vi "Easy Data.vi"() -> ()   [LabVIEW 2012]
doc: "This revision adds the ability to acquire data from a local computer running Dataserver software. It is also possible to type in the address for a new Dataserver computer that is not listed on the ceeserver webpage."
uses:
  support/method.ctl
  DataServer/command cluster.ctl
  DataServer/command.ctl
  DAQ configuration/Sensor array.ctl
  DAQ configuration/channel identifier.ctl
  toolbar icons/data not logging.ctl
  toolbar icons/open configuration.ctl
  DAQ configuration/stream state.ctl
  TCP DAQ/Set.ctl
  TCP DAQ/clear offset.ctl
  TCP DAQ/graph channel info.ctl
  toolbar icons/calibrator.ctl
  toolbar icons/log data.ctl
  toolbar icons/graph type.ctl
  TCP DAQ/zero.ctl
  toolbar icons/Data Source.ctl
  toolbar icons/help.ctl
  Process Controller 3.0/read-write.ctl
  Process Controller 3.0/ini interface.ctl
  DataServer/Server Stats.vi
  calibration/global scale array.vi
  <vilib>/Analysis/1siggen.llb/Ramp Pattern by Samples.vi
  <vilib>/Analysis/NI_AALBase.lvlib
panel:
  in  "Help":T1
  in  "Data Source":T2 caption="OK Button"
  in  "File Comment":bool
  in  "Freeze":bool
  in  "Clear":T3
  in  "Zero":T4
  in  "power user":bool
  out "XY Graph":T5(graph)
  in  "graph type":T6
  in  "Enable Logging data":T7
  in  "Calibrator":T8 caption="OK Button"
  out "digital display":dbl[](array[numeric]) format="%.2p"
  out "channel info":T9[](array[typedef])
  in  "calibration":T11(array[cluster])=[{"Set"=FALSE, "target value"=0.0, "Clear"=FALSE}, {"Set"=FALSE, "target value"=0.0, "Clear"=FALSE}, {"Set"=FALSE, "target value"=0.0, "Clear"=FALSE}, {"Set"=FALSE, "target value"=0.0, "Clear"=FALSE}, {"Set"=FALSE, "target value"=0.0, "Clear"=FALSE}, {"Set"=FALSE, "target value"=0.0, "Clear"=FALSE}, {"Set"=FALSE, "target value"=0.0, "Clear"=FALSE}, {"Set"=FALSE, "target value"=0.0, "Clear"=FALSE}, {"Set"=FALSE, "target value"=0.0, "Clear"=FALSE}, {"Set"=FALSE, "target value"=0.0, "Clear"=FALSE}, {"Set"=FALSE, "target value"=0.0, "Clear"=FALSE}, {"Set"=FALSE, "target value"=0.0, "Clear"=FALSE}] {"target value" format="%.1p"}
  in  "reset interval":dbl=1.0 min=1.0 format="%.1f"
  out "New Stream state":T12
  out "Stream state":T12
  in  "Display update frequency":ext=1.0 format="%.4f"
  out "Sampling data frequency":dbl
  in  "Open Configuration":T13
  out "file warning":T14
  in  "Sensor Array":T15
  out "scans acquired":u32
  out "seconds":u32
  out "data server address":string="calcium"
  in  "method":T17={"sampling interval"=0.1, "samples to average"=1, "data interval"=0.0, "stream data"=FALSE, "file path"=refnum, "command"={"command"=enum."Idle", "start time (ms)"=0, "Channel Indices"=[], "Scans per Sample"=1}} {"command"."Scans per Sample" min=1; "data interval" format="%.2f"; "samples to average" min=1 step=1; "sampling interval" format="%.2f"}
  in  "Data log status":bool
  in  "colors":u32[](array[colorbox])=[16711680, 16770090, 6487897, 16777215, 16753241, 16738047, 52479, 2556143, 16711680, 16770090, 7470980, 16777215, 16753241, 16738047, 52479, 2556143]
  out "error":errorcluster={"status"=FALSE, "code"=56, "source"="TCP Read in \u0000TCP read variable.vi->read Volts data fast.vi->Signal Monitor"}
  out "chart":sgl[][](graph)
  out "connection ID":refnum<k5>
  out "stop":bool=TRUE
  out "logging data to file:":path=path "C:/WINNT/Profiles/mlws/Desktop/50Hzjunk"
  # "current \nvalue"
  # "plot\ncolor"
  # "name"
  # "units"
  # "F1 toggles power user features"
  # "s"
  # "s"
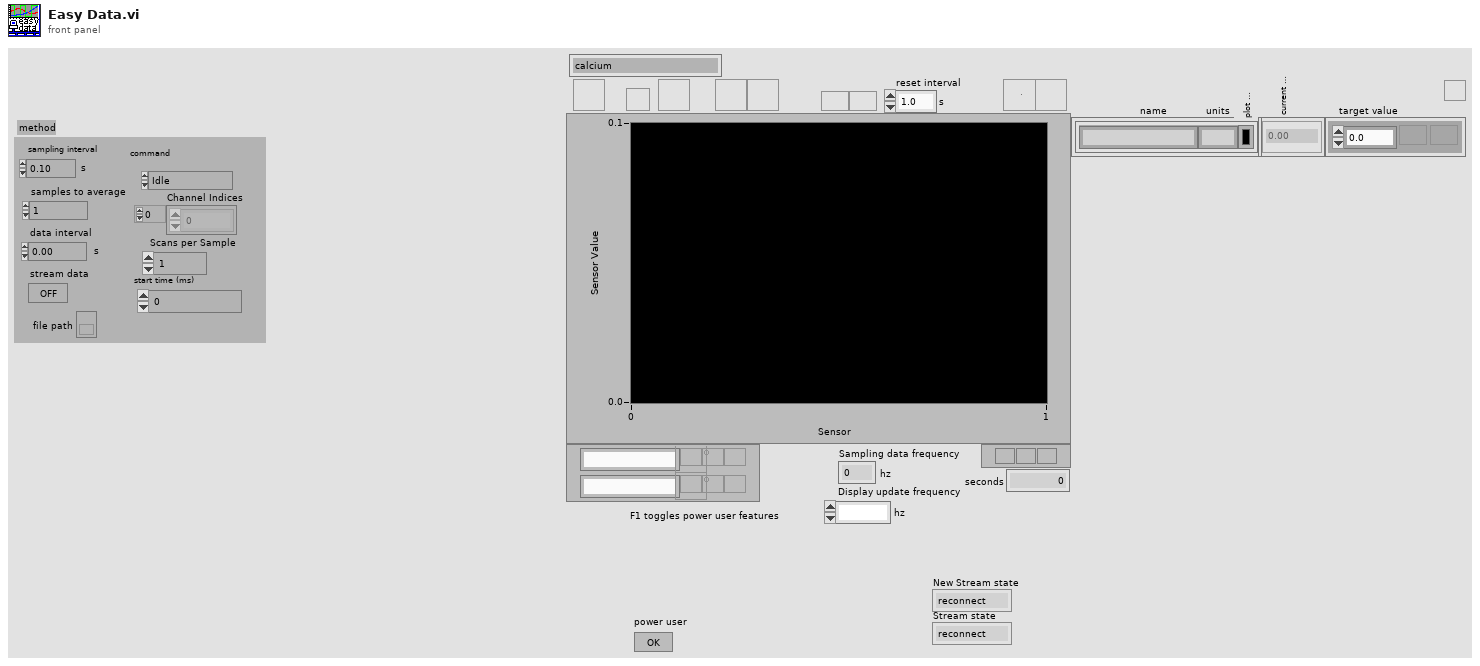
[diagram p1: front panel]
types:
  T1 = typedef "help.ctl" = bool
  T2 = typedef "Data Source.ctl" = bool
  T3 = typedef "clear offset.ctl" = bool
  T4 = typedef "zero.ctl" = bool
  T5 = cluster{"Ramp Pattern":dbl[], "last reading":sgl[]}
  T6 = typedef "graph type.ctl" = bool
  T7 = typedef "log data.ctl" = bool
  T8 = typedef "calibrator.ctl" = bool
  T9 = typedef "graph channel info.ctl" = cluster{"name":string, "units":string, "Color":u32}
  T10 = typedef "Set.ctl" = bool
  T11 = cluster{"Set":T10, "target value":dbl, "Clear":T3}[]
  T12 = typedef "stream state.ctl" = enum16{"reconnect", "Start", "Stream", "Clear", "Stop", "idle"}
  T13 = typedef "open configuration.ctl" = bool
  T14 = typedef "data not logging.ctl" = bool
  T15 = typedef "Sensor array.ctl" = T16[]
  T16 = typedef "channel identifier.ctl" = u16
  T17 = typedef "method.ctl" = cluster{"sampling interval":sgl, "samples to average":u32, "data interval":sgl, "stream data":bool, "file path":refnum<file>, "command":T18}
  T18 = typedef "command cluster.ctl" = cluster{"command":T19, "start time (ms)":u32, "Channel Indices":i32[], "Scans per Sample":i32}
  T19 = typedef "command.ctl" = enum16{"Idle", "Send Data", "Send 1 Scan", "Logoff"}
  T20 = typedef "ini interface.ctl" = enum16{"dataserver list", "dataserver", "com port", "stamp model", "Local Daq"}
  T21 = typedef "read-write.ctl" = enum16{"read", "write"}
  T22 = enum16{"Idle", "Send Data", "Send 1 Scan", "Logoff"}
  T23 = cluster{"Set":T10, "target value":dbl, "Clear":T3}
  T24 = typedef "Server stats.ctl" = cluster{"scan rate":dbl, "# connections":i32, "channel settings":cluster{"Name":string, "upper input limits":sgl, "lower input limits":sgl, "Location":string}[]}
  T25 = typedef "calib array.ctl" = T26[]
  T26 = typedef "conversion.ctl" = cluster{"conversion matrix":sgl[][], "units":string, "name":string, "scale type":T27, "offset (volts)":dbl, "second channel":i8, "correspondence table":T28, "offset (physical units)":dbl, "pH scale":T29, "D.O.":T30}
  T27 = typedef "scale type.ctl" = enum16{"Volts", "Polynomial", "Correspondence Table", "pH", "Dissolved Oxygen", "Quadratic"}
  T28 = typedef "correspondence table.ctl" = cluster{"physical units":dbl, "volts":dbl}[]
  T29 = typedef "pH scale.ctl" = cluster{"Buffers":cluster{"Buffer":dbl, "Calibrated":bool, "V/T":dbl}[], "Temperature":dbl}
  T30 = typedef "DO scale.ctl" = cluster{"Temperature":dbl, "K":dbl, "barometric pressure":dbl}
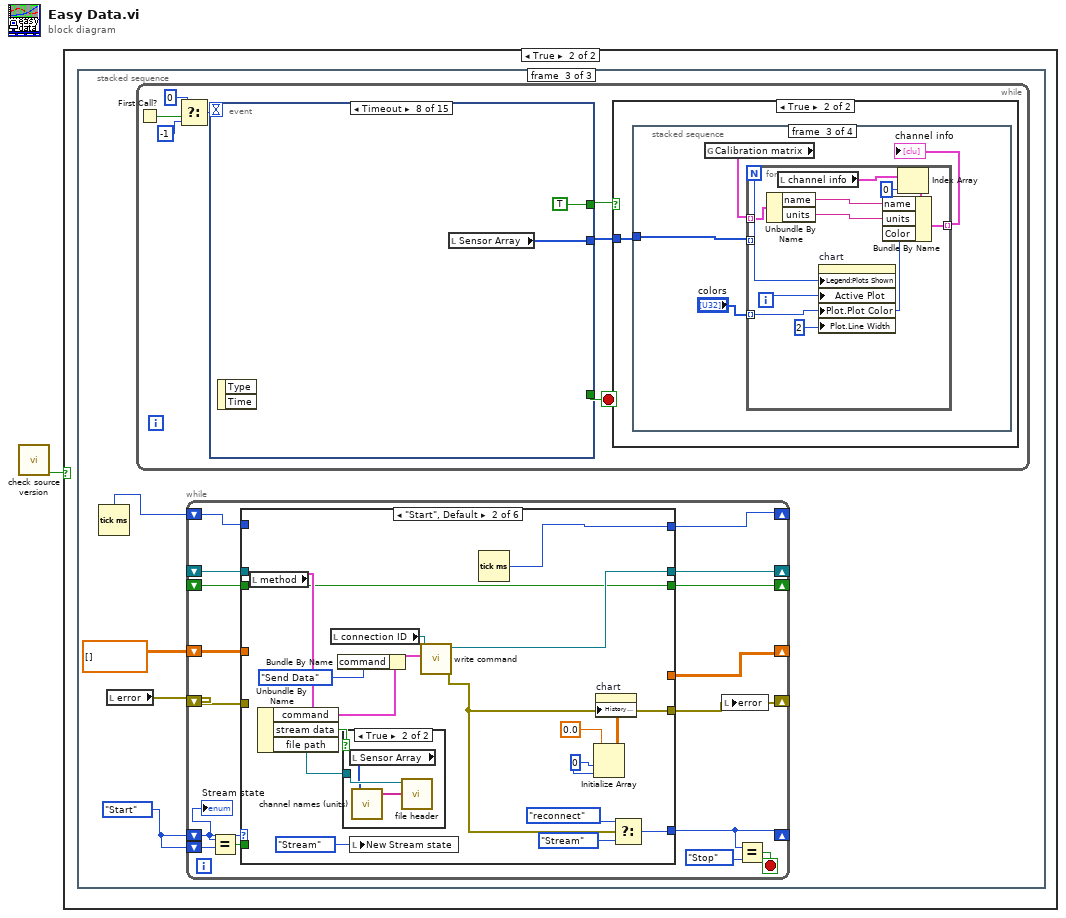
[diagram p0: block diagram]
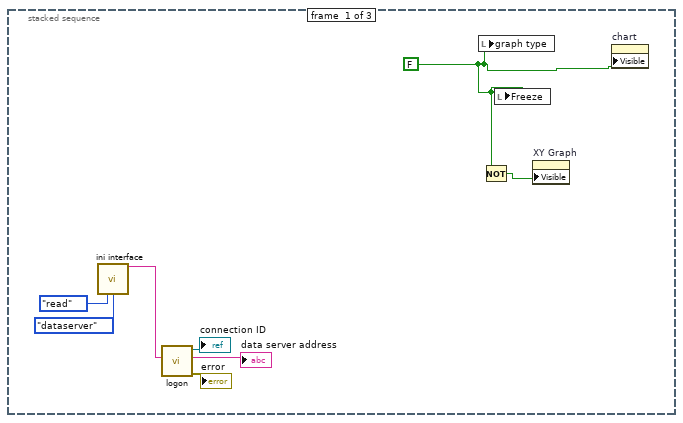
[diagram p3: hidden frame]
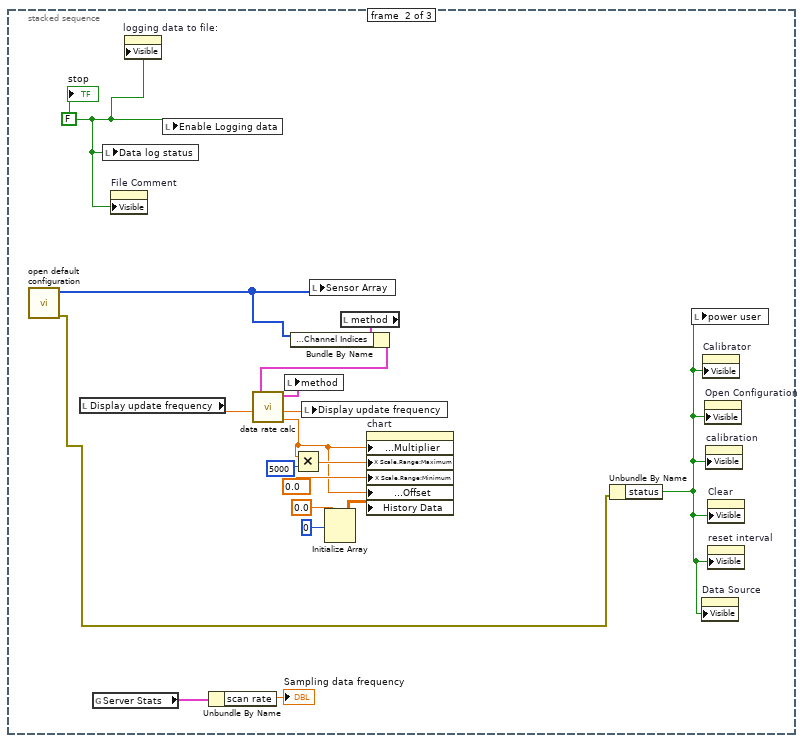
[diagram p4: hidden frame]
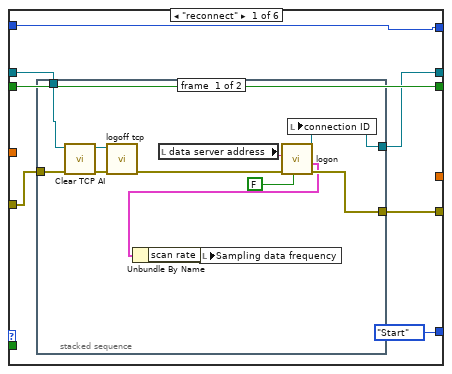
[diagram p5: hidden frame]
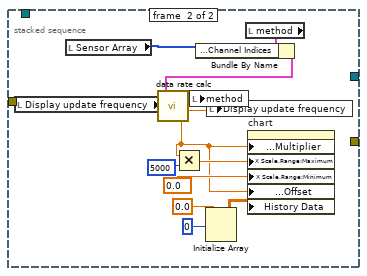
[diagram p6: hidden frame]
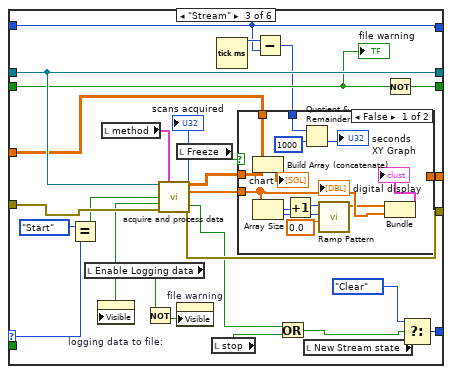
[diagram p8: hidden frame]
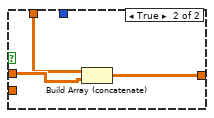
[diagram p9: hidden frame]
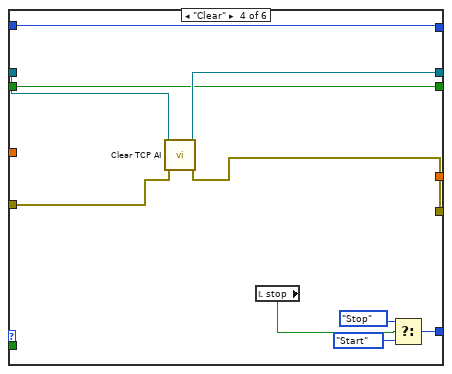
[diagram p10: hidden frame]
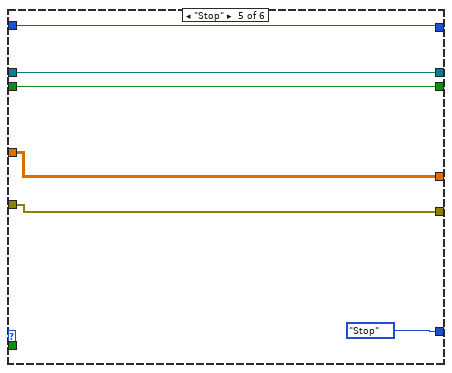
[diagram p11: hidden frame]
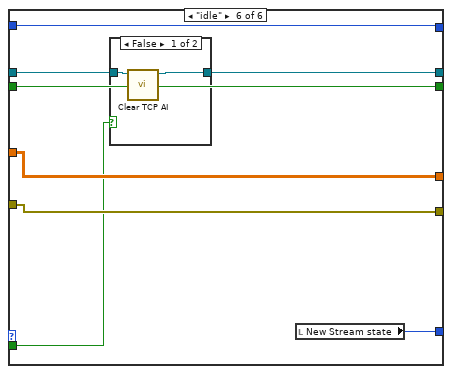
[diagram p12: hidden frame]
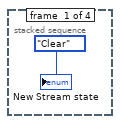
[diagram p15: hidden frame]
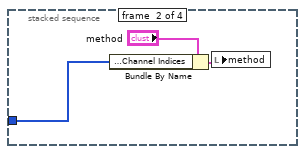
[diagram p16: hidden frame]
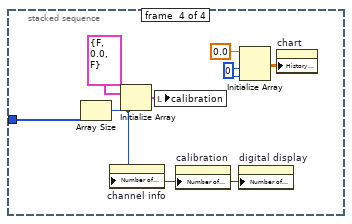
[diagram p17: hidden frame]
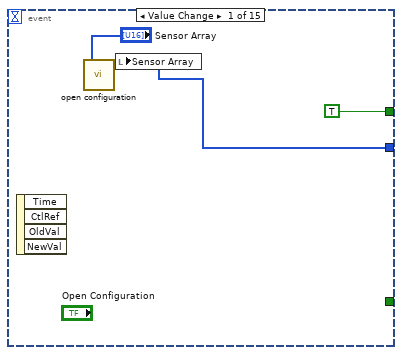
[diagram p18: hidden frame]
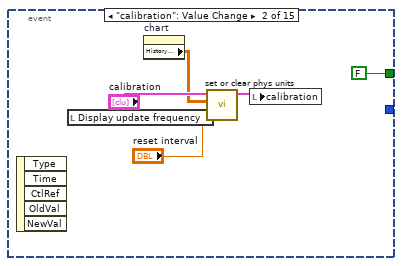
[diagram p19: hidden frame]
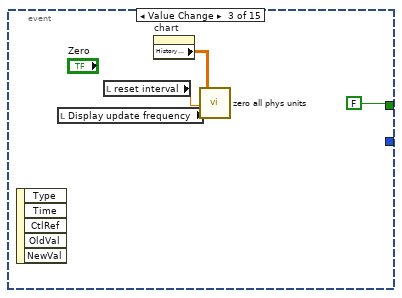
[diagram p20: hidden frame]
diagram:
  n1 = call "check source version.vi"() -> ("continue running?"=w1:bool)  [unwired: 2 in, 3 out]
  n2 = case shown="True" w1 {
    frame False {
    }
    frame True {
      n3 = stacked-sequence {
        frame #0 {
          w8 = T6 FALSE ("graph type")
          n4 = call "ini interface.vi"("direction"=read-write."read", "ini interface"=ini_interface."dataserver") -> ("dataserver out"=w2:string)  [unwired: 9 in, 4 out]
          n5 = call "logon.vi"("data server address in"=w2) -> ("error out"=→"error":errorcluster, "data server address"=→"data server address":string, "connection ID"=→"connection ID":refnum<k5>)  [unwired: 7 in, 1 out]
          n6 = local write "graph type"(w8) -> ()
          n7 = Not(x=w8) -> (.not. x?=w9:T6)
          n8 = local write "Freeze"(w8) -> ()
          n9 = property on="XY Graph" class="XYGraph (strict)"("Visible"=w9) -> ()  [unwired: 2 in, 2 out]
          n10 = property on="chart" class="WFChart (strict)"("Visible"=w8) -> ()  [unwired: 2 in, 2 out]
        }
        frame #1 {
          w23 = 0
          w25 = FALSE
          n11 = call "open default configuration.vi"() -> ("error out"=w12:errorcluster, "Sensor Array out"=w10:T15)  [unwired: 6 in]
          n12 = local read "Display update frequency"() -> (w14:ext)
          n13 = global read "Server Stats.vi" "Server Stats"() -> (w27:T24)
          n14 = local write "Data log status"(w25) -> ()
          n15 = property on="File Comment" class="Bool"("Visible"=w25) -> ()  [unwired: 2 in, 2 out]
          n16 = property on="logging data to file:" class="Path"("Visible"=w25) -> ()  [unwired: 2 in, 2 out]
          n17 = local write "Enable Logging data"(w25) -> ()
          n18 = Unbundle By Name(w27) -> ("scan rate"=→"Sampling data frequency":dbl)
          n19 = local write "Sensor Array"(w10) -> ()
          n20 = Initialize Array(sgl 0.0, w23, w23) -> (w17:sgl[][])
          n21 = local read "method"() -> (w16:T17)
          n22 = Bundle By Name(cluster=w16, "command.Channel Indices"=w10) -> (w15:T17)
          n23 = call "data rate calc.vi"("Data frequency"=w14, "method in"=w15) -> ("new data interval"=w18:sgl, "new data frequency"=w13:ext, "method out"=w19:T17)  [unwired: 2 in, 1 out]
          n24 = local write "method"(w19) -> ()
          n25 = Multiply(x=w18, y=5000) -> (x*y=w21:sgl)
          n26 = local write "Display update frequency"(w13) -> ()
          n27 = property on="chart" class="WFChart (strict)"("X Scale.Offset and Multiplier:Multiplier"=w18, "X Scale.Range:Maximum"=w21, "X Scale.Range:Minimum"=0.0, "X Scale.Offset and Multiplier:Offset"=w18, "History Data"=w17) -> ()  [unwired: 2 in, 2 out]
          n28 = Unbundle By Name(w12) -> ("status"=w11:bool)
          n29 = local write "power user"(w11) -> ()
          n30 = property on="Data Source" class="Bool"("Visible"=w11) -> ()  [unwired: 2 in, 2 out]
          n31 = property on="Calibrator" class="Bool"("Visible"=w11) -> ()  [unwired: 2 in, 2 out]
          n32 = property on="Open Configuration" class="Bool"("Visible"=w11) -> ()  [unwired: 2 in, 2 out]
          n33 = property on="calibration" class="Arr"("Visible"=w11) -> ()  [unwired: 2 in, 2 out]
          n34 = property on="Clear" class="Bool"("Visible"=w11) -> ()  [unwired: 2 in, 2 out]
          n35 = property on="reset interval" class="DigNum (strict)"("Visible"=w11) -> ()  [unwired: 2 in, 2 out]
          "stop" <- w25
        }
        frame #2 {
          w28 = stream_state."Start" ("Stream state")
          n36 = Tick Count (ms)() -> (millisecond timer value=w29:u32)
          n37 = local read "error"() -> (w31:errorcluster)
          n38 = while {
            stop <- w174 stop-if-true
            n39 = First Call?() -> (First Call?: T/F=w169:bool)
            n40 = Select(t=0, s=w169, f=-1) -> (s? t:f=w168:i32)
            n41 = event shown="[7] Timeout" {
              selector: _ -> [_ _ _ _ _ _ _ _ _ _ _ _ _ _ _]
              dyn-events: _ -> [_ _ _ _ _ _ _ _ _ _ _ _ _ _ _]
              timeout: w168 -> [_ _ _ _ _ _ _ _ _ _ _ _ _ _ _]
              tunnel: [_ _ _ _ _ _ w224 _ _ _ _ _ _ _ w293] -> w174
              tunnel: [w203 _ _ _ w218 _ _ w229 w231 _ _ _ _ _ _] -> w173
              tunnel: [TRUE FALSE FALSE _ TRUE _ w224 TRUE TRUE FALSE FALSE FALSE _ _ FALSE] -> w172
              event Value Change {
                n42 = event-data() -> ()  [unwired: 1 in, 4 out]
                n43 = call "open configuration.vi"("Sensor Array"="Sensor Array") -> ("Sensor Array out"=w203:T15)  [unwired: 5 in, 1 out]
                n44 = local write "Sensor Array"(w203) -> ()
              }
              event "calibration": Value Change {
                n45 = event-data() -> ()  [unwired: 1 in, 5 out]
                n46 = local read "Display update frequency"() -> (w208:ext)
                n47 = property on="chart" class="WFChart (strict)"() -> ("History Data"=w205:sgl[][])  [unwired: 2 in, 2 out]
                n48 = call "set or clear phys units.vi"("zero interval (s)"="reset interval", "Data frequency"=w208, "History Data"=w205, "calibration"="calibration") -> ("calibration out"=w207:T11)  [unwired: 3 in]
                n49 = local write "calibration"(w207) -> ()
              }
              event Value Change {
                n50 = event-data() -> ()  [unwired: 1 in, 5 out]
                n51 = local read "Display update frequency"() -> (w213:ext)
                n52 = local read "reset interval"() -> (w212:dbl)
                n53 = property on="chart" class="WFChart (strict)"() -> ("History Data"=w211:sgl[][])  [unwired: 2 in, 2 out]
                n54 = call "zero all phys units.vi"("zero interval (s)"=w213, "Data frequency"=w212, "History Data"=w211) -> ()  [unwired: 5 in]
              }
              event Value Change {
                n55 = event-data() -> ()  [unwired: 1 in, 5 out]
                n56 = local read "Sensor Array"() -> (w215:T15)
                n57 = for {
                  tunnel: w215 -> [_] mode=indexing
                  i -> [w216]
                  n58 = call "clear channel physical units.vi"("Index"=w216) -> ()  [unwired: 7 in]
                }
              }
              event Value Change {
                n59 = event-data() -> ()  [unwired: 1 in, 5 out]
                n60 = stacked-sequence {
                  tunnel: [_ w221] -> w218
                  frame #0 {
                    n61 = local write "New Stream state"(stream_state."idle" ("New Stream state")) -> ()
                  }
                  frame #1 {
                    n62 = local read "Sensor Array"() -> (w222:T15)
                    n63 = local read "data server address"() -> (w220:string)
                    n64 = call "Calibrator.vi"("data server address"=w220, "Channels"=w222) -> ("Ports out"=w221:T15)  [unwired: 6 in, 2 out]
                    n65 = local write "Sensor Array"(w221) -> ()
                  }
                }
              }
              event Value Change {
                n66 = event-data() -> ()  [unwired: 1 in, 6 out]
                n67 = call "Web Browser.vi"("URL"="http://ceeserver.cee.cornell.edu/mw24/Software/Easy Data.htm") -> ()  [unwired: 1 in]
              }
              event Value Change {
                w224 = FALSE
                n68 = event-data() -> ()  [unwired: 1 in, 6 out]
                n69 = stacked-sequence {
                  frame #0 {
                    n70 = call "Select server.vi"() -> ("DataSource"=w225:string)  [unwired: 5 in]
                    n71 = local write "data server address"(w225) -> ()
                    n72 = call "ini interface.vi"("dataserver"=w225, "direction"=read-write."write", "ini interface"=ini_interface."dataserver") -> ()  [unwired: 8 in, 5 out]
                  }
                  frame #1 {
                    n73 = local write "New Stream state"(stream_state."reconnect" ("New Stream state")) -> ()
                  }
                }
              }
              event Timeout {
                n74 = event-data() -> ()  [unwired: 1 in, 2 out]
                n75 = local read "Sensor Array"() -> (w229:T15)
              }
              event "Display update frequency": Value Change {
                w241 = 0
                n76 = event-data() -> ()  [unwired: 1 in, 5 out]
                n77 = local read "Sampling data frequency"() -> (w237:dbl)
                n78 = local read "method"() -> (w242:T17)
                n79 = In Range and Coerce(upper limit=w237, x="Display update frequency", lower limit=ext 0.01) -> (coerced(x)=w234:ext)  [unwired: 1 out]
                n80 = call "data rate calc.vi"("Data frequency"=w234, "method in"=w242) -> ("new data interval"=w233:sgl, "new data frequency"=w232:ext, "method out"=w243:T17)  [unwired: 2 in, 1 out]
                n81 = Initialize Array(w241, w241, w241) -> (w238:i32[][])
                n82 = local write "Display update frequency"(w232) -> ()
                n83 = Multiply(x=w233, y=5000) -> (x*y=w240:sgl)
                n84 = property on="chart" class="WFChart (strict)"("X Scale.Offset and Multiplier:Multiplier"=w233, "X Scale.Range:Maximum"=w240, "X Scale.Range:Minimum"=w241, "X Scale.Offset and Multiplier:Offset"=w233, "History Data"=w238) -> ()  [unwired: 2 in, 2 out]
                n85 = local write "method"(w243) -> ()
                n86 = local read "Sensor Array"() -> (w231:T15)
              }
              event Value Change {
                n87 = event-data() -> ()  [unwired: 1 in, 5 out]
                n88 = local read "Sensor Array"() -> (w245:T15)
                n89 = property on="file warning" class="Bool"("Visible"=FALSE) -> ()  [unwired: 2 in, 2 out]
                n90 = Not Equal?(x="Data log status", y="Enable Logging data") -> (x != y?=w250:T7)
                n91 = case shown="True" w250 {
                  tunnel: "Enable Logging data" -> [_ w252]
                  tunnel: w245 -> [_ w251]
                  frame False {
                  }
                  frame True {
                    n92 = case shown="True" w252 {
                      selector: w252 -> [w253 _]
                      tunnel: w251 -> [_ w258]
                      frame False {
                        n93 = local read "method"() -> (w255:T17)
                        n94 = local write "Data log status"(w253) -> ()
                        n95 = property on="logging data to file:" class="Path"("Visible"=w253) -> ()  [unwired: 2 in, 2 out]
                        n96 = Unbundle By Name(w255) -> ("file path"=w254:refnum<file>)
                        n97 = Bundle By Name(cluster=w255, "stream data"=w253, "file path"=refnum<k0> refnum) -> (w257:T17)
                        n98 = local write "method"(w257) -> ()
                        n99 = Close File(refnum=w254) -> ()  [unwired: 1 in, 2 out]
                        n100 = property on="File Comment" class="Bool"("Visible"=w253) -> ()  [unwired: 2 in, 2 out]
                      }
                      frame True {
                        n101 = call "Create xls File.vi"() -> ("error out"=w260:errorcluster, "path"=w259:path, "refnum"=w261:refnum<file>)  [unwired: 4 in, 1 out]
                        n102 = case shown="No Error" w260 {
                          tunnel: w261 -> [w264 _]
                          tunnel: w259 -> [w266 _]
                          tunnel: w258 -> [w262 _]
                          frame No Error {
                            n103 = Not A Number/Path/Refnum?(number/path/refnum=w264) -> (NaN/Path/Refnum?=w267:bool)
                            n104 = local read "method"() -> (w268:T17)
                            n105 = call "channel names (units).vi"("Sensor Array"=w262) -> ("channel strings"=w265:string[])  [unwired: 4 in]
                            n106 = Bundle By Name(cluster=w268, "stream data"=TRUE, "file path"=w264) -> (w269:T17)
                            n107 = Not(x=w267) -> (.not. x?=w263:bool)
                            n108 = local write "Enable Logging data"(w263) -> ()
                            n109 = local write "Data log status"(w263) -> ()
                            n110 = call "file header.vi"("channel strings"=w265, "refnum"=w264) -> ()  [unwired: 9 in, 1 out]
                            n111 = property on="logging data to file:" class="Path"("Visible"=w263) -> ()  [unwired: 2 in, 2 out]
                            n112 = local write "method"(w269) -> ()
                            n113 = property on="File Comment" class="Bool"("Visible"=w263) -> ()  [unwired: 2 in, 2 out]
                            "logging data to file:" <- w266
                          }
                          frame Error {
                            w271 = FALSE
                            n114 = local write "Enable Logging data"(w271) -> ()
                            n115 = local write "Data log status"(w271) -> ()
                            n116 = property on="logging data to file:" class="Path"("Visible"=w271) -> ()  [unwired: 2 in, 2 out]
                            n117 = property on="File Comment" class="Bool"("Visible"=w271) -> ()  [unwired: 2 in, 2 out]
                          }
                        }
                      }
                    }
                  }
                }
              }
              event Value Change {
                n118 = event-data() -> ()  [unwired: 1 in, 5 out]
                n119 = Not(x="graph type") -> (.not. x?=w272:T6)
                n120 = Not(x=w272) -> (.not. x?=w275:T6)
                n121 = property on="XY Graph" class="XYGraph (strict)"("Visible"=w272) -> ()  [unwired: 2 in, 2 out]
                n122 = property on="chart" class="WFChart (strict)"("Visible"=w275) -> ()  [unwired: 2 in, 2 out]
              }
              event "power user": Value Change {
                n123 = event-data() -> ()  [unwired: 1 in, 5 out]
                n124 = property on="calibration" class="Arr"("Visible"="power user") -> ()  [unwired: 2 in, 2 out]
                n125 = property on="Calibrator" class="Bool"("Visible"="power user") -> ()  [unwired: 2 in, 2 out]
                n126 = property on="Open Configuration" class="Bool"("Visible"="power user") -> ()  [unwired: 2 in, 2 out]
                n127 = property on="Clear" class="Bool"("Visible"="power user") -> ()  [unwired: 2 in, 2 out]
                n128 = property on="reset interval" class="DigNum (strict)"("Visible"="power user") -> ()  [unwired: 2 in, 2 out]
                n129 = property on="Data Source" class="Bool"("Visible"="power user") -> ()  [unwired: 2 in, 2 out]
              }
              event "Freeze": Value Change {
                w280 = u32 1535
                n130 = event-data() -> ()  [unwired: 1 in, 5 out]
                n131 = Select(t=w280, s="Freeze", f=u32 13816530) -> (s? t:f=w279:u32)
                n132 = Select(t=u32 16448250, s="Freeze", f=u32 0) -> (s? t:f=w281:u32)
                n133 = Select(t=w280, s="Freeze", f=u32 0) -> (s? t:f=w278:u32)
                n134 = property on="seconds" class="DigNum (strict)"("Numeric Text.Text Colors:BG Color"=w279, "Numeric Text.Text Colors:Text Color"=w281) -> ()  [unwired: 2 in, 2 out]
                n135 = property on="current value" class="DigNum (strict)"("Numeric Text.Text Colors:BG Color"=w279, "Numeric Text.Text Colors:Text Color"=w281) -> ()  [unwired: 2 in, 2 out]
                n136 = property on="XY Graph" class="XYGraph (strict)"("Plot Area:Colors:BG Color"=w278) -> ()  [unwired: 2 in, 2 out]
                n137 = property on="chart" class="WFChart (strict)"("Plot Area:Colors:BG Color"=w278) -> ()  [unwired: 2 in, 2 out]
              }
              event "File Comment": Value Change {
                n138 = event-data() -> ()  [unwired: 1 in, 5 out]
                n139 = local read "method"() -> (w288:T17)
                n140 = Unbundle By Name(w288) -> ("file path"=w287:refnum<file>)
                n141 = call "Write comment to file.vi"("refnum"=w287) -> ()  [unwired: 7 in, 2 out]
              }
              event Application Instance Close? {
                w293 = TRUE ("Quit")
                n142 = event-data() -> ()  [unwired: 1 in, 2 out]
                n143 = local read "connection ID"() -> (w292:refnum<k5>)
                n144 = local read "method"() -> (w290:T17)
                n145 = Unbundle By Name(w290) -> ("file path"=w291:refnum<file>)
                n146 = call "logoff tcp.vi"("Connection ID"=w292) -> ()  [unwired: 9 in, 2 out]
                n147 = local write "stop"(w293) -> ()
                n148 = Close File(refnum=w291) -> ()  [unwired: 1 in, 2 out]
                n149 = event-data() -> ()  [unwired: 2 in, 1 out]
              }
            }
            n150 = case shown="True" w172 {
              tunnel: w173 -> [_ w175]
              frame False {
              }
              frame True {
                n151 = stacked-sequence {
                  tunnel: w175 -> [_ w177 w181 w196]
                  frame #0 {
                    "New Stream state" <- stream_state."Clear" ("Stream state")
                  }
                  frame #1 {
                    n152 = Bundle By Name(cluster="method", "command.Channel Indices"=w177) -> (w178:T17)
                    n153 = local write "method"(w178) -> ()
                  }
                  frame #2 {
                    n154 = global read "global scale array.vi" "Calibration matrix"() -> (w182:T25)
                    n155 = for {
                      N -> [w193]
                      tunnel: [w192] -> w183 mode=indexing
                      tunnel: w182 -> [w189] mode=indexing
                      tunnel: w181 -> [_] mode=indexing
                      tunnel: "colors" -> [w185] mode=indexing
                      i -> [w194]
                      n156 = Unbundle By Name(w189) -> ("name"=w191:string, "units"=w190:string)
                      n157 = local read "channel info"() -> (w188:T9[])
                      n158 = property on="chart" class="WFChart (strict)"("Legend:Plots Shown"=w193, "Active Plot"=w194, "Plot.Plot Color"=w185, "Plot.Line Width"=u8 2) -> ()  [unwired: 2 in, 2 out]
                      n159 = Index Array(array=w188, index=0) -> (element=w186:T9)
                      n160 = Bundle By Name(cluster=w186, "name"=w191, "units"=w190, "Color"=w185) -> (w192:T9)
                    }
                    "channel info" <- w183
                  }
                  frame #3 {
                    w201 = 0
                    n161 = Array Size(array=w196) -> (size(s)=w195:i32)
                    n162 = property on="channel info" class="Arr (strict)"("Number of Rows"=w195) -> ()  [unwired: 2 in, 2 out]
                    n163 = Initialize Array(T23 {"Set"=FALSE, "target value"=0.0, "Clear"=FALSE} ("Cluster"), w195) -> (w198:T11)
                    n164 = local write "calibration"(w198) -> ()
                    n165 = property on="calibration" class="Arr"("Number of Rows"=w195) -> ()  [unwired: 2 in, 2 out]
                    n166 = property on="digital display" class="Arr (strict)"("Number of Rows"=w195) -> ()  [unwired: 2 in, 2 out]
                    n167 = Initialize Array(sgl 0.0, w201, w201) -> (w199:sgl[][])
                    n168 = property on="chart" class="WFChart (strict)"("History Data"=w199) -> ()  [unwired: 2 in, 2 out]
                  }
                }
              }
            }
          }
          n169 = while {
            shift-left: _ -> [w46]
            shift-right: [w44] -> _
            shift-right: [w40] -> _
            shift-left: w31 -> [w47]
            shift-right: [w43] -> _
            shift-right: [w42] -> _
            shift-left: _ -> [w41]
            shift-left: w28 -> [w33]
            shift-right: [w39] -> _
            shift-left: sgl[][] [] -> [w38]
            shift-right: [w37] -> _
            shift-left: w29 -> [w36]
            shift-left: w28 -> [w34]
            stop <- w45 stop-if-true
            n170 = Equal?(x=w33, y=w34) -> (x = y?=w32:bool)
            n171 = case shown="\"Start\", Default" w33 {
              selector: w33 -> [_ _ w112 _ _ _]
              tunnel: [w50 w85 w123 w145 w155 w161] -> w43
              tunnel: w47 -> [w49 _ w125 w150 w155 w161]
              tunnel: w46 -> [w52 _ w124 w149 w152 w159]
              tunnel: [w51 w87 w124 w148 w152 w158] -> w44
              tunnel: [stream_state."Start" ("Stream state") w84 w122 w147 stream_state."Stop" ("Stream state") w160] -> w40
              tunnel: [w54 w83 w121 w146 w153 w163] -> w42
              tunnel: w41 -> [w54 w83 w108 w146 w153 w163]
              tunnel: [_ _ w106 _ w154 w162] -> w39
              tunnel: w38 -> [_ _ w105 _ w154 w162]
              tunnel: [w53 w82 w102 w143 w151 w164] -> w37
              tunnel: w36 -> [w53 _ w102 w143 w151 w164]
              tunnel: w32 -> [_ _ _ _ _ w157]
              frame "reconnect" {
                n172 = stacked-sequence {
                  tunnel: w52 -> [w65 _]
                  tunnel: [w59 _] -> w51
                  tunnel: [w60 _] -> w50
                  tunnel: w49 -> [w62 _]
                  frame #0 {
                    n173 = call "Clear TCP AI.vi"("error in (no error)"=w62, "Connection ID in"=w65) -> ("error out"=w63:errorcluster, "Connection ID out"=w64:refnum<k5>)  [unwired: 8 in]
                    n174 = call "logoff tcp.vi"("error in (no error)"=w63, "Connection ID"=w64) -> ("error out"=w58:errorcluster)  [unwired: 8 in, 1 out]
                    n175 = local read "data server address"() -> (w61:string)
                    n176 = call "logon.vi"("Display error messages?"=FALSE, "error in"=w58, "data server address in"=w61) -> ("error out"=w60:errorcluster, "Server stats"=w56:T24, "connection ID"=w59:refnum<k5>)  [unwired: 5 in, 1 out]
                    n177 = Unbundle By Name(w56) -> ("scan rate"=w57:dbl)
                    n178 = local write "Sampling data frequency"(w57) -> ()
                    n179 = local write "connection ID"(w59) -> ()
                  }
                  frame #1 {
                    w77 = 0
                    n180 = local read "Display update frequency"() -> (w68:ext)
                    n181 = local read "Sensor Array"() -> (w66:T15)
                    n182 = Initialize Array(sgl 0.0, w77, w77) -> (w71:sgl[][])
                    n183 = local read "method"() -> (w70:T17)
                    n184 = Bundle By Name(cluster=w70, "command.Channel Indices"=w66) -> (w69:T17)
                    n185 = call "data rate calc.vi"("Data frequency"=w68, "method in"=w69) -> ("new data interval"=w72:sgl, "new data frequency"=w67:ext, "method out"=w73:T17)  [unwired: 2 in, 1 out]
                    n186 = Multiply(x=w72, y=5000) -> (x*y=w75:sgl)
                    n187 = local write "method"(w73) -> ()
                    n188 = local write "Display update frequency"(w67) -> ()
                    n189 = property on="chart" class="WFChart (strict)"("X Scale.Offset and Multiplier:Multiplier"=w72, "X Scale.Range:Maximum"=w75, "X Scale.Range:Minimum"=0.0, "X Scale.Offset and Multiplier:Offset"=w72, "History Data"=w71) -> ()  [unwired: 2 in, 2 out]
                  }
                }
              }
              frame "Start", Default {
                w91 = 0
                n190 = local read "method"() -> (w95:T17)
                n191 = Unbundle By Name(w95) -> ("command"=w92:T18, "stream data"=w93:bool, "file path"=w94:refnum<file>)
                n192 = local read "connection ID"() -> (w86:refnum<k5>)
                n193 = Bundle By Name(cluster=w92, "command"=T22."Send Data") -> (w96:T18)
                n194 = case shown="True" w93 {
                  tunnel: w94 -> [_ w99]
                  frame False {
                  }
                  frame True {
                    n195 = local read "Sensor Array"() -> (w97:T15)
                    n196 = call "channel names (units).vi"("Sensor Array"=w97) -> ("channel strings"=w98:string[])  [unwired: 4 in]
                    n197 = call "file header.vi"("channel strings"=w98, "refnum"=w99) -> ()  [unwired: 9 in, 1 out]
                  }
                }
                n198 = local write "New Stream state"(stream_state."Stream" ("Stream state")) -> ()
                n199 = call "write command.vi"("command interface"=w96, "refnum in"=w86) -> ("error out"=w85:errorcluster, "refnum out"=w87:refnum<k5>)  [unwired: 8 in]
                n200 = Tick Count (ms)() -> (millisecond timer value=w82:u32)
                n201 = Initialize Array(sgl 0.0, w91, w91) -> (w89:sgl[][])
                n202 = property on="chart" class="WFChart (strict)"("History Data"=w89) -> ()  [unwired: 2 in, 2 out]
                n203 = Select(t=stream_state."reconnect" ("Stream state"), s=w85, f=stream_state."Stream" ("Stream state")) -> (s? t:f=w84:T12)
              }
              frame "Stream" {
                n204 = Equal?(x=stream_state."Start" ("Stream state"), y=w112) -> (x = y?=w117:bool)
                n205 = local read "Enable Logging data"() -> (w120:T7)
                n206 = property on="logging data to file:" class="Path"("Visible"=w120) -> ()  [unwired: 2 in, 2 out]
                n207 = local read "method"() -> (w118:T17)
                n208 = Not(x=w120) -> (.not. x?=w119:T7)
                n209 = call "acquire and process data.vi"("connection ID"=w124, "Reset"=w117, "Log Data"=w120, "error in"=w125, "method"=w118) -> ("samples"=→"scans acquired":u32, "data out"=w107:sgl[][], "last reading"=w110:sgl[], "Status"=w115:bool, "error out"=w123:errorcluster)  [unwired: 3 in, 3 out]
                n210 = local read "Freeze"() -> (w109:bool)
                n211 = property on="file warning" class="Bool"("Visible"=w119) -> ()  [unwired: 2 in, 2 out]
                n212 = local read "stop"() -> (w116:bool)
                n213 = Tick Count (ms)() -> (millisecond timer value=w104:u32)
                n214 = Subtract(x=w104, y=w102) -> (x-y=w103:u32)
                n215 = case shown="False" w109 {
                  tunnel: w110 -> [w136 _]
                  tunnel: w107 -> [w130 w140]
                  tunnel: [_ w139] -> w106
                  tunnel: w105 -> [w131 w138]
                  tunnel: w103 -> [w126 _]
                  frame False {
                    n216 = Build Array (concatenate)(w131, w130) -> (→"chart":sgl[][])
                    n217 = Array Size(array=w136) -> (size(s)=w134:i32)
                    n218 = Increment(x=w134) -> (x+1=w135:i32)
                    n219 = Quotient & Remainder(x=w126, y=u32 1000) -> (floor(x/y)=→"seconds":u32)  [unwired: 1 out]
                    n220 = call-poly <vilib>:"Ramp Pattern.vi"("start"=0.0, "end"=w134, "samples"=w135) -> ("Ramp Pattern"=w133:dbl[])  [unwired: 7 in, 1 out]
                    n221 = Bundle("Ramp Pattern"=w133, "last reading"=w136) -> (→"XY Graph":T5)  [unwired: 1 in]
                    "digital display" <- w136
                  }
                  frame True {
                    n222 = Build Array (concatenate)(w138, w140) -> (w139:sgl[][])
                  }
                }
                n223 = Or(x=w115, y=w116) -> (x .or. y?=w114:bool)
                n224 = local read "New Stream state"() -> (w113:T12)
                n225 = Not(x=w108) -> (.not. x?=w121:bool)
                n226 = Select(t=stream_state."Clear" ("Stream state"), s=w114, f=w113) -> (s? t:f=w122:T12)
                "file warning" <- w108
              }
              frame "Clear" {
                n227 = call "Clear TCP AI.vi"("error in (no error)"=w150, "Connection ID in"=w149) -> ("error out"=w145:errorcluster, "Connection ID out"=w148:refnum<k5>)  [unwired: 8 in]
                n228 = local read "stop"() -> (w144:bool)
                n229 = Select(t=stream_state."Stop" ("Stream state"), s=w144, f=stream_state."Start" ("Stream state")) -> (s? t:f=w147:T12)
              }
              frame "Stop" {
              }
              frame "idle" {
                n230 = case shown="False" w157 {
                  tunnel: w159 -> [w166 w167]
                  tunnel: [w165 w167] -> w158
                  frame False {
                    n231 = call "Clear TCP AI.vi"("Connection ID in"=w166) -> ("Connection ID out"=w165:refnum<k5>)  [unwired: 9 in, 1 out]
                  }
                  frame True {
                  }
                }
                n232 = local read "New Stream state"() -> (w160:T12)
              }
            }
            n233 = local write "error"(w43) -> ()
            n234 = Equal?(x=w40, y=stream_state."Stop" ("Stream state")) -> (x = y?=w45:bool)
            "Stream state" <- w33
          }
        }
      }
    }
  }
